vi "Display Unicode Strings on Graph and Chart.vi"() -> ()   [LabVIEW 2009]
uses:
  _subVIs/tool_Unicode_Convert ASCII to Unicode (Scalar).vi
panel:
  in  "Caption":string="My Unicode Chart"
  out "Waveform Chart":dbl(graph)
  in  "Caption":string="My Unicode Graph"
  out "error out":errorcluster
  in  "Y Axis Label":string
  in  "X Axis Label":string
  out "Waveform Graph":dbl[](graph)
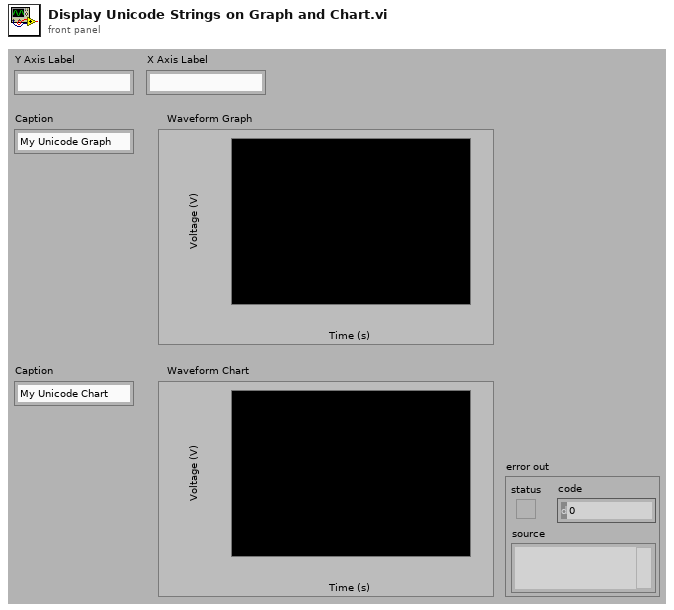
[diagram p1: front panel]
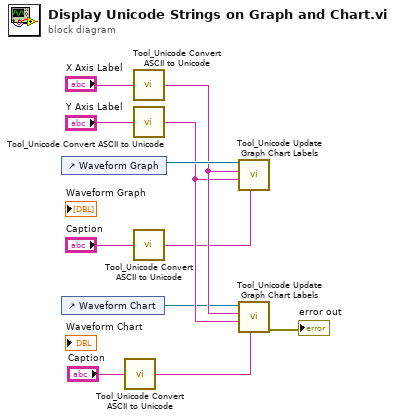
[diagram p0: block diagram]
diagram:
  n1 = control-ref of="Waveform Graph"() -> (w7:refnum<vi>)
  n2 = control-ref of="Waveform Chart"() -> (w3:refnum<vi>)
  n3 = call-poly "Tool_Unicode Convert ASCII to Unicode.vi"("ASCII"="Caption") -> ("Unicode"=w2:string)  [unwired: 4 in]
  n4 = call-poly "Tool_Unicode Convert ASCII to Unicode.vi"("ASCII"="X Axis Label") -> ("Unicode"=w6:string)  [unwired: 4 in]
  n5 = call-poly "Tool_Unicode Convert ASCII to Unicode.vi"("ASCII"="Y Axis Label") -> ("Unicode"=w5:string)  [unwired: 4 in]
  n6 = call-poly "Tool_Unicode Convert ASCII to Unicode.vi"("ASCII"="Caption") -> ("Unicode"=w4:string)  [unwired: 4 in]
  n7 = call "Tool_Unicode Update Graph Chart Labels.vi"("Caption"=w4, "Y Axis Label"=w5, "X Axis Label"=w6, "GrphChrt Ref"=w7) -> ()  [unwired: 6 in, 2 out]
  n8 = call "Tool_Unicode Update Graph Chart Labels.vi"("Caption"=w2, "Y Axis Label"=w5, "X Axis Label"=w6, "GrphChrt Ref"=w3) -> ("error out"=→"error out":errorcluster)  [unwired: 6 in, 1 out]
